vi "子VI-缺陷面积和Z值筛选.vi"(8 "计入缺陷的Z值阈值":i32, 9 "计入分层缺陷的面积阈值":i32, 11 "分层测量结果":dbl[][](array[numeric])) -> (2 "初始化的数组":dbl[][](array[numeric]), 3 "去掉的面积累计":dbl)   [LabVIEW 2018]
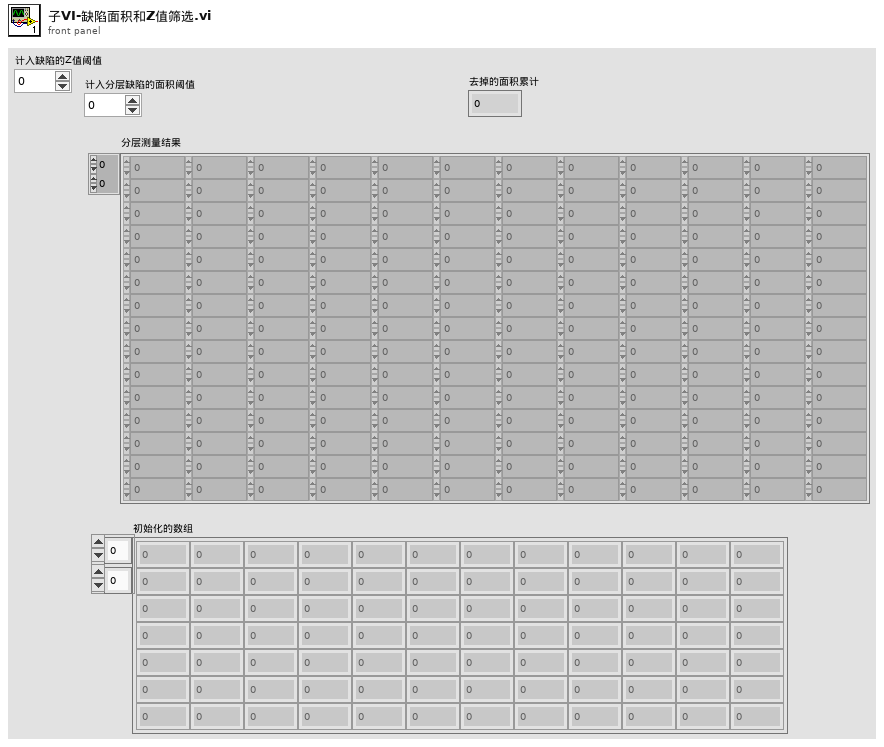
[diagram p1: front panel]
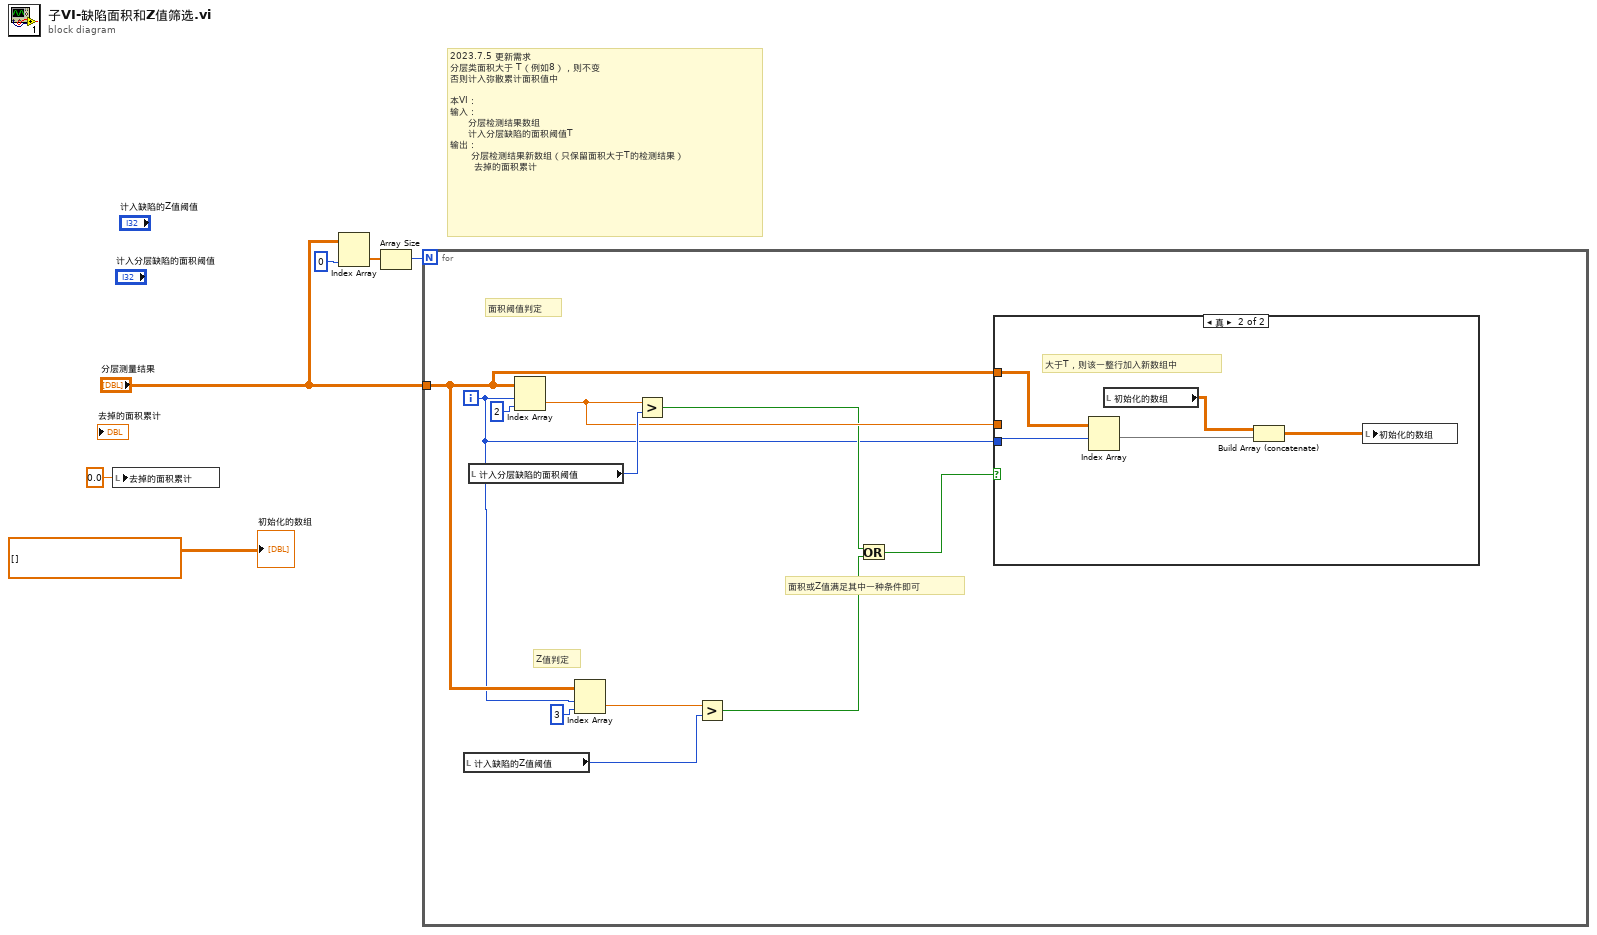
[diagram p0: block diagram]
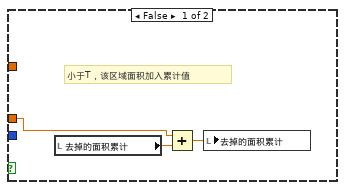
[diagram p2: hidden frame]
diagram:
  # "2023.7.5 更新需求\n分层类面积大于 T（例如8），则不变\n否则计入弥散累计面积值中\n\n本VI：\n输入：\n      分层检测结果数组\n      计入分层缺陷的面积阈值T\n输出：\n       分层检测结果新数组（只保留面积大于T的检测结果）\n        去掉的面积累计"
  n1 = local write "去掉的面积累计"(0.0 ("去掉的面积累计")) -> ()
  n2 = Index Array(array="分层测量结果", index (col)=0 ("禁用的索引 (列)")) -> (element=w4:dbl[])  [unwired: 1 in]
  n3 = Array Size(array=w4) -> (size(s)=w5:i32)
  n4 = for {
    N: w5 -> [_]
    tunnel: "分层测量结果" -> [w10]
    i -> [w9]
    # "面积或Z值满足其中一种条件即可"
    # "面积阈值判定"
    # "Z值判定"
    n5 = local read "计入缺陷的Z值阈值"() -> (w7:i32)
    n6 = local read "计入分层缺陷的面积阈值"() -> (w16:i32)
    n7 = Index Array(array=w10, index (row)=w9, index (col)=2 ("索引 (列)")) -> (element=w15:dbl)
    n8 = Index Array(array=w10, index (row)=w9, index (col)=3 ("索引 (列)")) -> (element=w8:dbl)
    n9 = Greater?(x=w15, y=w16) -> (0:w13:bool)
    n10 = Greater?(x=w8, y=w7) -> (0:w12:bool)
    n11 = Or(x=w13, y=w12) -> (x .or. y?=w11:bool)
    n12 = case shown="真" w11 {
      tunnel: w15 -> [w18 _]
      tunnel: w9 -> [_ w21]
      tunnel: w10 -> [_ w25]
      frame False {
        # "小于T，该区域面积加入累计值"
        n13 = local read "去掉的面积累计"() -> (w19:dbl)
        n14 = Add(x=w18, y=w19) -> (x+y=w20:dbl)
        n15 = local write "去掉的面积累计"(w20) -> ()
      }
      frame True {
        # "大于T，则该一整行加入新数组中"
        n16 = Index Array(array=w25, index (row)=w21) -> (element=w24:dbl[])  [unwired: 1 in]
        n17 = local read "初始化的数组"() -> (w23:dbl[][])
        n18 = Build Array (concatenate)(w23, w24) -> (w22:dbl[][])
        n19 = local write "初始化的数组"(w22) -> ()
      }
    }
  }
  "初始化的数组" <- dbl[][] [] ("初始化的数组")
